vi "Scalar_Data_2.vi"() -> ()   [LabVIEW 2012]
panel:
  out "Scalar Data 2":u16[](array[numeric])
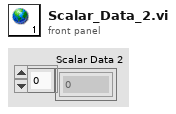
[diagram p1: front panel]
diagram:
